vi "Main.vi"() -> ()   [LabVIEW 2017]
doc: "This sample project is built upon the standard state machine template and shows how you could create an application that acquires, analyzes, and presents data. It includes functionality for presenting configuration dialogs, preserving settings between executions, loading and saving data, as well as exporting graph images and text files.\n\nIt is most appropriate for data that is acquired instantly as it does not allow for screen updates mid acquisition nor does it allow for continuous streaming to disk."
uses:
  controls/State.ctl
  controls/UI References.ctl
  controls/Graph Data.ctl
  <vilib>/Utility/miscctls.llb/LVAnnotationListTypeDef.ctl
  <vilib>/Utility/miscctls.llb/LVCursorListTypeDef.ctl
  controls/User Specified Data.ctl
  controls/HW Configuration.ctl
  controls/Analysis Configuration.ctl
  controls/New Data Behavior.ctl
  controls/Signal Configuration.ctl
panel:
  in  "Settings":bool
  in  "Snapshot":bool
  in  "Analyze":bool
  in  "Clear":bool
  in  "Exit":bool
  in  "Acquire":bool
  in  "Export":bool
  in  "Save Data":bool
  in  "Load Data":bool
  in  "Tab Control":enum32{"Data", "FFT Magnitude", "FFT Phase"}(tab)
  out "Data Graph":waveform(dbl)[](graph)
  out "FFT Magnitude":cluster{"f0":dbl, "df":dbl, "magnitude":dbl[]}[](graph)
  out "FFT Phase":cluster{"f0":dbl, "df":dbl, "magnitude":dbl[]}[](graph)
  out "Status Bar":string
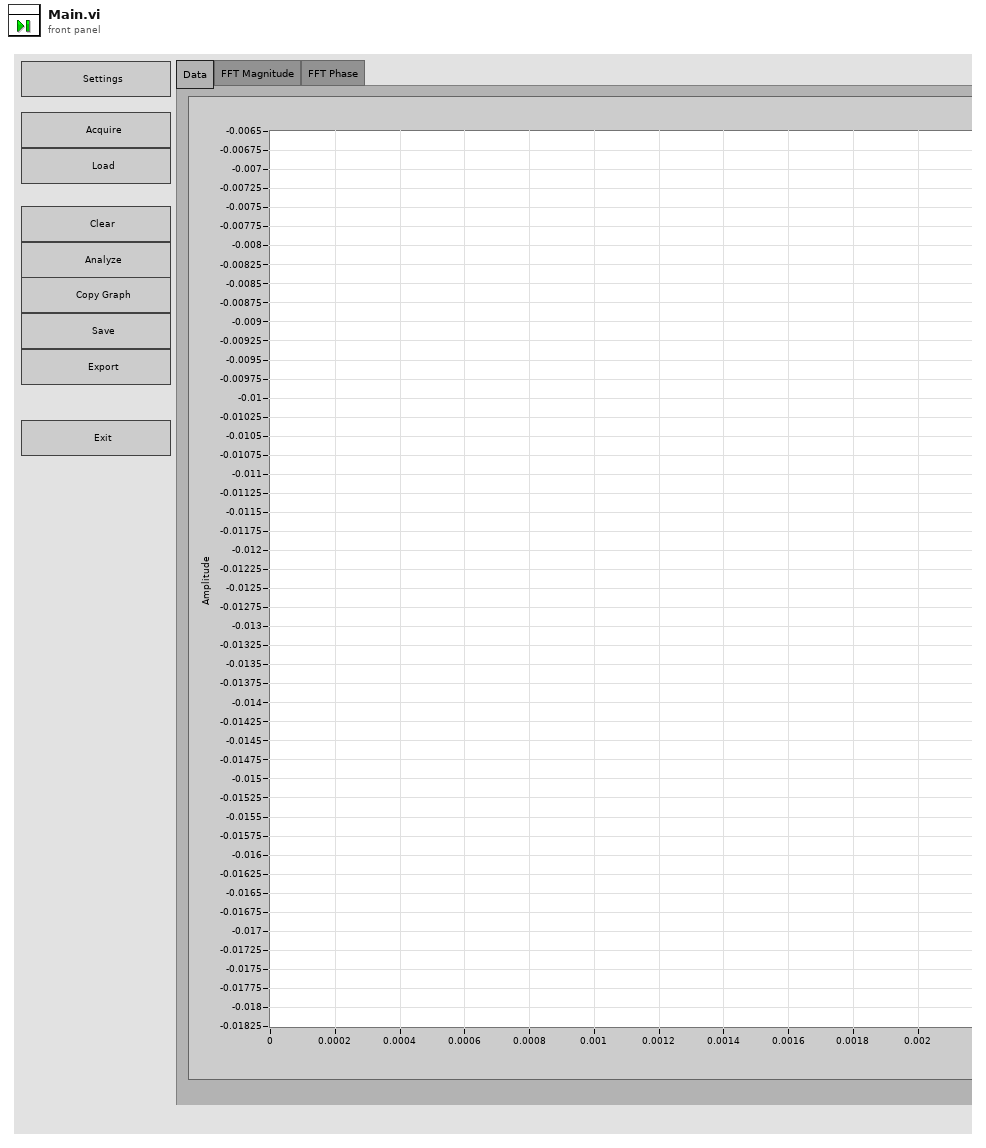
[diagram p1: front panel]
types:
  T1 = typedef "UI References.ctl" = cluster{"Stop Ref":refnum<vi>, "Save Ref":refnum<vi>, "Open Ref":refnum<vi>, "Export Ref":refnum<vi>, "Acquire Ref":refnum<vi>, "Configure Ref":refnum<vi>, "Graph Ref":refnum<vi>, "Clear Ref":refnum<vi>, "Analyze Ref":refnum<vi>, "Status Ref":refnum<vi>, "Snapshot Ref":refnum<vi>}
  T2 = typedef "Graph Data.ctl" = cluster{"Data":waveform(dbl)[], "Annotation List":T3, "Cursor List":T4, "Analysis Data":waveform(dbl)[]}
  T3 = typedef "LVAnnotationListTypeDef.ctl" = cluster{"Name":string, "Color":u32, "Style":u8, "Point Style":u8, "Name Visible":bool, "Allow Drag":bool, "Annotation Mode":u32, "Plot":i32, "Index":i32, "Position":cluster{"X":dbl, "Y":dbl}, "X Scale":u32, "Y Scale":u32, "Show Arrow":bool, "Lock Name":bool, "Plot Area":i32, "Label Offset":cluster{"X":dbl, "Y":dbl}}[]
  T4 = typedef "LVCursorListTypeDef.ctl" = cluster{"Name":string, "Color":u32, "Style":u8, "Point Style":u8, "Name Visible":bool, "Allow Drag":bool, "Cursor Mode":u32, "Plot":i32, "Index":i32, "Position":cluster{"X":dbl, "Y":dbl}, "X Scale":u32, "Y Scale":u32, "Watch Plots":i32[], "Watch All Plots":bool, "Plot Area":i32, "Label Offset":cluster{"X":dbl, "Y":dbl}}[]
  T5 = typedef "User Specified Data.ctl" = cluster{"Hardware Configuration":T6, "Analysis Configuration":T7, "Signal Type":enum16{"Single Chirp", "From Excel"}, "New Data Behavior":T8, "Signal Configuration":T9}
  T6 = typedef "HW Configuration.ctl" = cluster{"Signal Channel":tag, "Response Channel":tag, "Trigger Channel":tag, "Number of acquisitions":dbl}
  T7 = typedef "Analysis Configuration.ctl" = cluster{"Statistics":bool}
  T8 = typedef "New Data Behavior.ctl" = enum16{"Replace", "Overlay", "Append"}
  T9 = typedef "Signal Configuration.ctl" = cluster{"Chirp Amplitude":dbl, "I/O Limit":dbl, "Sample Rate":dbl, "Chirp Duration (s)":dbl, "Upper Frequency":dbl, "Lower Frequency":dbl, "Windowing":enum16{"None", "Exponential", "Flat top", "Hamming", "Hanning", "Kaiser-Bessel", "Rectangular"}}
  T10 = cluster{"UI References":T1, "Graph Data":T2, "User Specified":T5}
  T11 = typedef "State.ctl" = enum16{"Initialize", "Wait for Event", "Update UI", "Configure", "Acquire", "Load Data", "Save Data", "Clear Data", "Export Data", "Analyze", "Copy Graph", "Exit"}
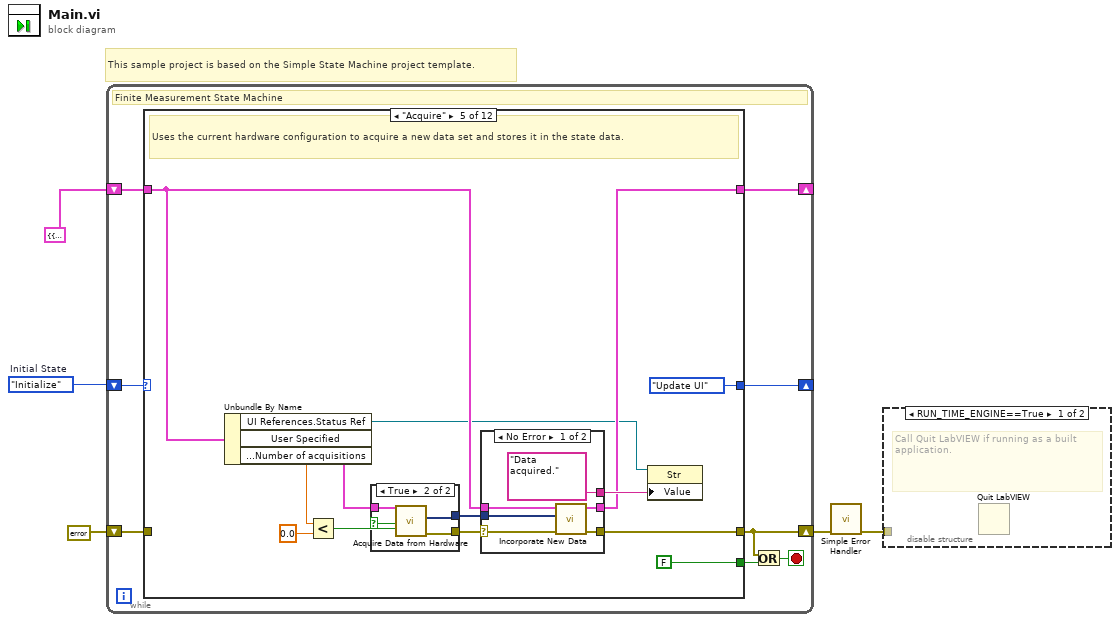
[diagram p0: block diagram]
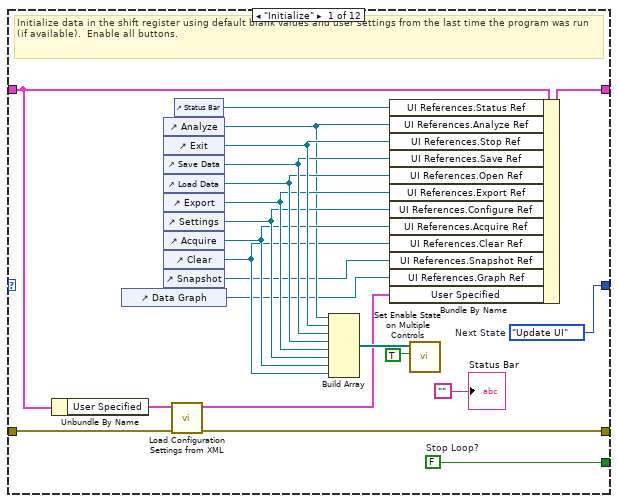
[diagram p3: hidden frame]
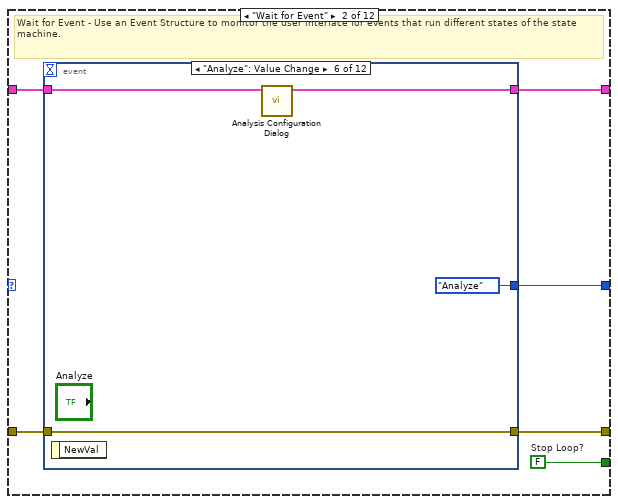
[diagram p4: hidden frame]
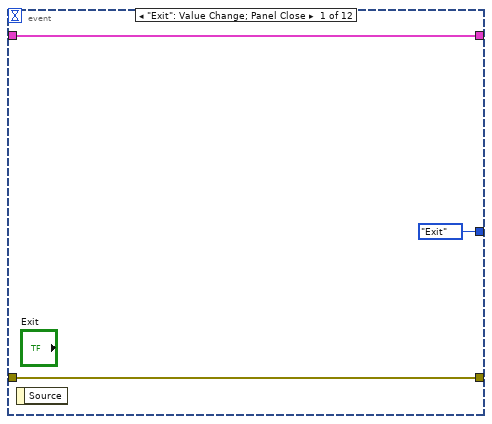
[diagram p5: hidden frame]
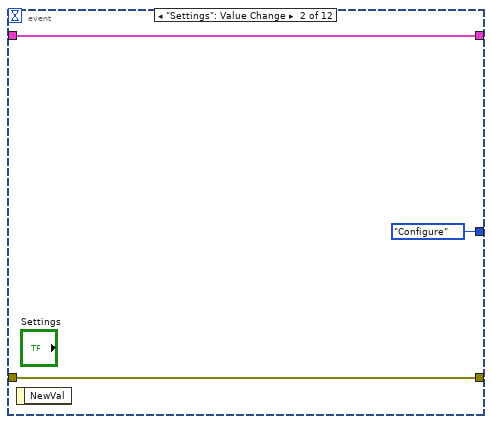
[diagram p6: hidden frame]
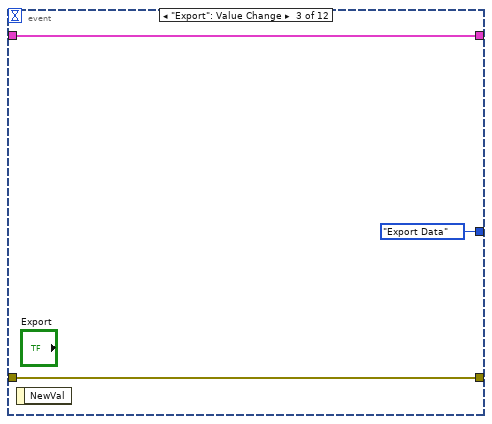
[diagram p7: hidden frame]
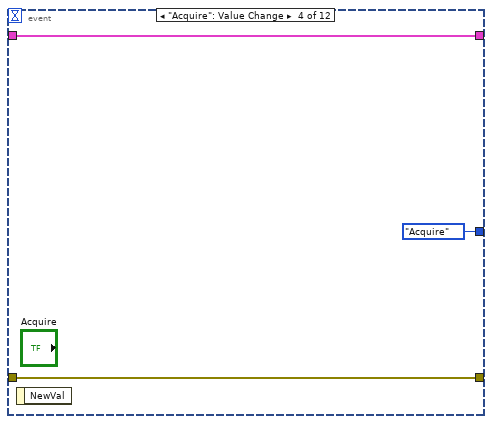
[diagram p8: hidden frame]
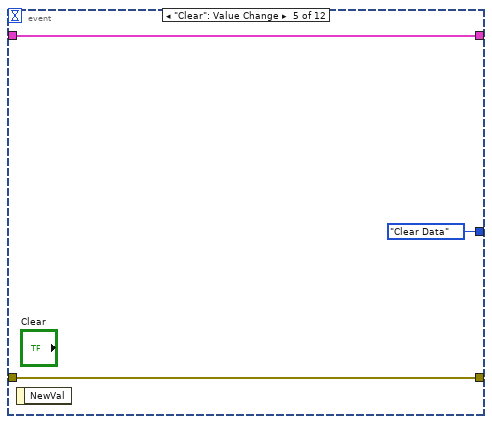
[diagram p9: hidden frame]
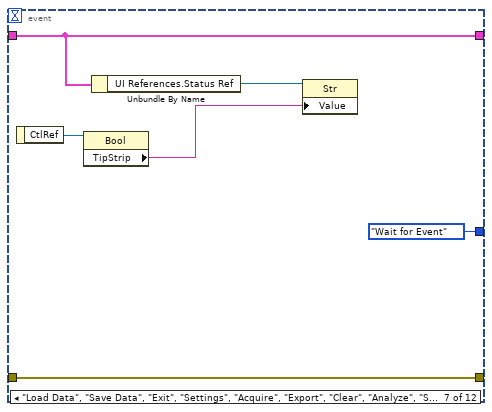
[diagram p10: hidden frame]
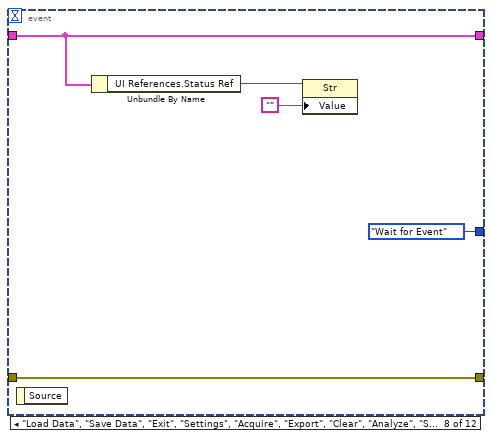
[diagram p11: hidden frame]
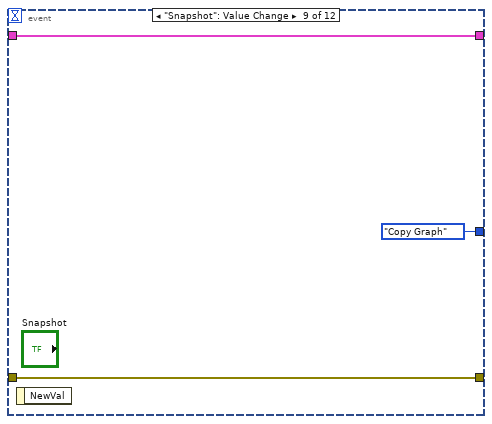
[diagram p12: hidden frame]
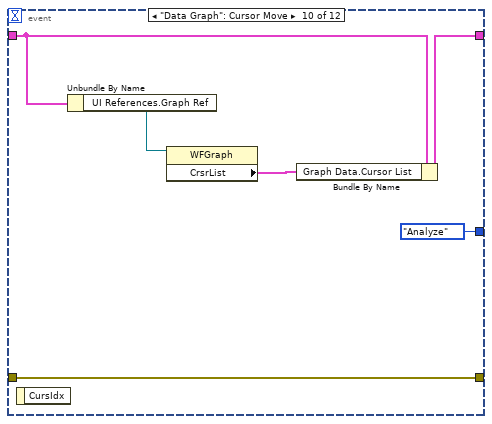
[diagram p13: hidden frame]
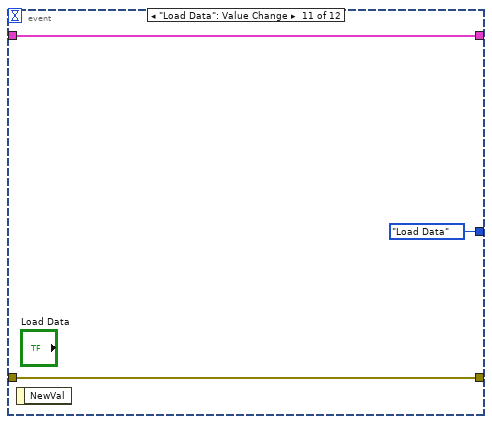
[diagram p14: hidden frame]
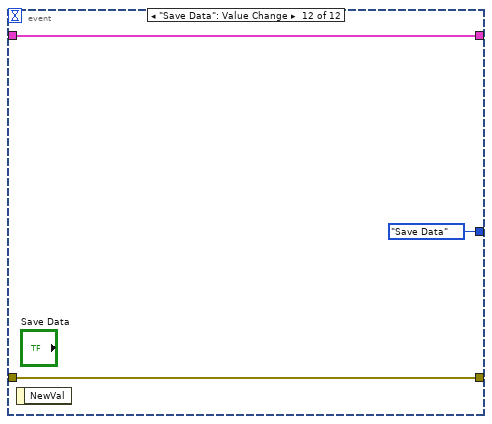
[diagram p15: hidden frame]
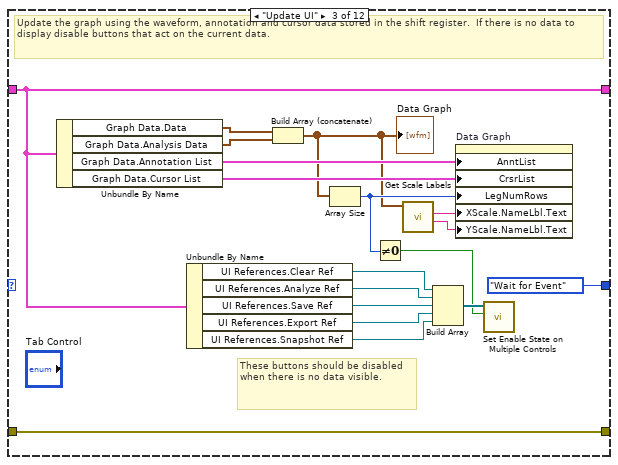
[diagram p16: hidden frame]
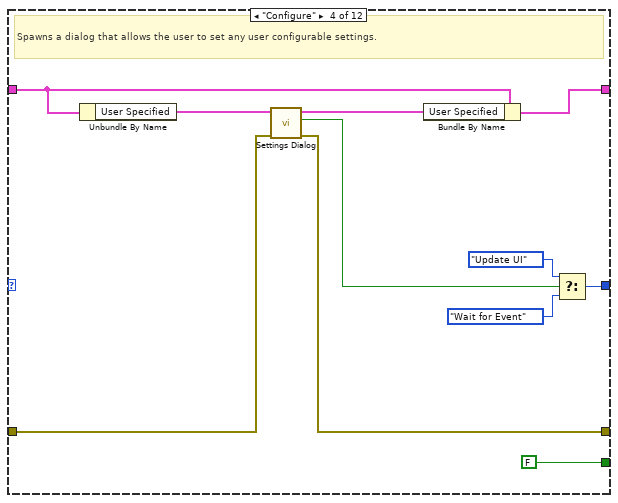
[diagram p17: hidden frame]
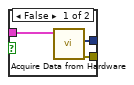
[diagram p18: hidden frame]
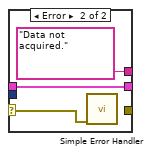
[diagram p19: hidden frame]
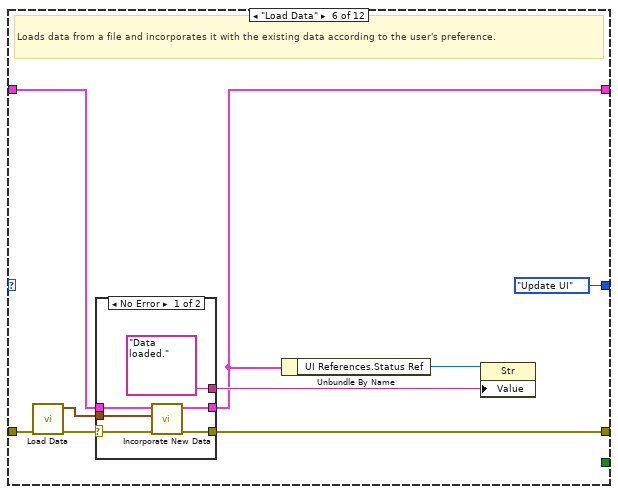
[diagram p20: hidden frame]
diagram:
  w5 = State."Initialize"  # Initial State
  # "This sample project is based on the Simple State Machine project template."
  n1 = while {
    shift-right: [w12] -> _
    shift-left: w5 -> [w13]
    shift-right: [w10] -> _
    shift-left: T10 {"UI References"={"Stop Ref"=refnum, "Save Ref"=refnum, "Open Ref"=refnum, "Export Ref"=refnum, "Acquire Ref"=refnum, "Configure Ref"=refnum, "Graph Ref"=refnum, "Clear Ref"=refnum, "Analyze Ref"=refnum, "Status Ref"=refnum, "Snapshot Ref"=refnum}, "Graph Data"={"Data"=[], "Annotation List"=[], "Cursor List"=[], "Analysis Data"=[]}, "User Specified"={"Hardware Configuration"={"Signal Channel"="", "Response Channel"="", "Trigger Channel"="", "Number of acquisitions"=0.0}, "Analysis Configuration"={"Statistics"=FALSE}, "Signal Type"=enum."Single Chirp", "New Data Behavior"=enum."Replace", "Signal Configuration"={"Chirp Amplitude"=0.1, "I/O Limit"=10.0, "Sample Rate"=1000000.0, "Chirp Duration (s)"=10000000.0, "Upper Frequency"=0.0, "Lower Frequency"=0.0, "Windowing"=enum."None"}}} ("Data") -> [w11]
    shift-right: [w6] -> w2
    shift-left: errorcluster {"status"=FALSE, "code"=0, "source"=""} ("error constant") -> [w9]
    stop <- w7 stop-if-true
    # "Finite Measurement State Machine"
    n2 = case shown="\"Acquire\"" w13 {
      tunnel: [w35 w41 State."Wait for Event" ("(Value Not Used)") w108 State."Update UI" ("Next State") State."Update UI" ("(Value Not Used)") State."Wait for Event" ("(Value Not Used)") State."Wait for Event" ("(Value Not Used)") State."Update UI" ("(Value Not Used)") State."Update UI" ("(Value Not Used)") State."Wait for Event" ("(Value Not Used)") w208] -> w12
      tunnel: [w34 w40 _ FALSE ("Stop Loop?") FALSE ("Stop Loop?") _ _ _ _ _ _ w207] -> w8
      tunnel: w11 -> [w25 w39 w101 w114 w124 w152 w165 w174 w187 w193 w197 w205]
      tunnel: [w33 w38 w101 w113 w123 w146 w165 w174 w186 w193 w197 w205] -> w10
      tunnel: w9 -> [w23 w37 w104 w112 _ w151 w167 w179 w189 w195 w199 w202]
      tunnel: [w22 w36 w104 w111 w119 w150 w163 w175 w189 w195 w198 w201] -> w6
      frame "Initialize" {
        w34 = FALSE  # Stop Loop?
        w35 = State."Update UI"  # Next State
        # "Initialize data in the shift register using default blank values and user settings from the last time the program was run (if available).  Enable all buttons."
        n3 = Unbundle By Name(w25) -> ("User Specified"=w24:T5)
        n4 = control-ref of="Data Graph"() -> (w14:refnum<vi>)
        n5 = control-ref of="Analyze"() -> (w21:refnum<vi>)
        n6 = control-ref of="Exit"() -> (w32:refnum<vi>)
        n7 = control-ref of="Save Data"() -> (w31:refnum<vi>)
        n8 = control-ref of="Load Data"() -> (w30:refnum<vi>)
        n9 = control-ref of="Export"() -> (w29:refnum<vi>)
        n10 = control-ref of="Settings"() -> (w28:refnum<vi>)
        n11 = control-ref of="Acquire"() -> (w27:refnum<vi>)
        n12 = control-ref of="Clear"() -> (w19:refnum<vi>)
        n13 = control-ref of="Snapshot"() -> (w15:refnum<vi>)
        n14 = call "Load Configuration Settings from XML.vi"("error in (no error)"=w23, "User Configuration in"=w24) -> ("error out"=w22:errorcluster, "User Configuration out"=w17:T5)  [unwired: 8 in]
        n15 = control-ref of="Status Bar"() -> (w20:refnum<vi>)
        n16 = Build Array(w21, w32, w31, w30, w29, w28, w27, w19) -> (w26:refnum<vi>[])
        n17 = Bundle By Name(cluster=w25, "UI References.Status Ref"=w20, "UI References.Analyze Ref"=w21, "UI References.Stop Ref"=w32, "UI References.Save Ref"=w31, "UI References.Open Ref"=w30, "UI References.Export Ref"=w29, "UI References.Configure Ref"=w28, "UI References.Acquire Ref"=w27, "UI References.Clear Ref"=w19, "UI References.Snapshot Ref"=w15, "UI References.Graph Ref"=w14, "User Specified"=w17) -> (w33:T10)
        n18 = call "Set Enable State on Multiple Controls.vi"("Enable?"=TRUE, "Controls"=w26) -> ()  [unwired: 10 in]
        "Status Bar" <- "" ("Status Bar")
      }
      frame "Wait for Event" {
        w40 = FALSE  # Stop Loop?
        # "Wait for Event - Use an Event Structure to monitor the user interface for events that run different states of the state machine."
        n19 = event shown="[5] \"Analyze\": Value Change" {
          selector: _ -> [_ _ _ _ _ _ _ _ _ _ _ _]
          dyn-events: _ -> [_ _ _ _ _ _ _ _ _ _ _ _]
          timeout: _ -> [_ _ _ _ _ _ _ _ _ _ _ _]
          tunnel: [State."Exit" ("Next State") State."Configure" ("Next State") State."Export Data" ("Next State") State."Acquire" ("Next State") State."Clear Data" ("Next State") State."Analyze" ("Next State") State."Wait for Event" ("Next State") State."Wait for Event" ("Next State") State."Copy Graph" ("Next State") State."Analyze" ("Next State") State."Load Data" ("Next State") State."Save Data" ("Next State")] -> w41
          tunnel: w39 -> [w43 w47 w50 w53 w56 w58 w64 w70 w74 w75 w82 w85]
          tunnel: [w43 w47 w50 w53 w56 w57 w64 w70 w74 w78 w82 w85] -> w38
          tunnel: w37 -> [w42 w46 w49 w52 w55 w60 w66 w71 w73 w80 w81 w84]
          tunnel: [w42 w46 w49 w52 w55 w60 w66 w71 w73 w80 w81 w84] -> w36
          event "Exit": Value Change; Panel Close {
            n20 = event-data() -> ()  [unwired: 1 in, 1 out]
          }
          event "Settings": Value Change {
            n21 = event-data() -> ()  [unwired: 1 in, 1 out]
          }
          event "Export": Value Change {
            n22 = event-data() -> ()  [unwired: 1 in, 1 out]
          }
          event "Acquire": Value Change {
            n23 = event-data() -> ()  [unwired: 1 in, 1 out]
          }
          event "Clear": Value Change {
            n24 = event-data() -> ()  [unwired: 1 in, 1 out]
          }
          event "Analyze": Value Change {
            n25 = event-data() -> ()  [unwired: 1 in, 1 out]
            n26 = call "Analysis Configuration Dialog.vi"("Data in"=w58) -> ("Data out"=w57:T10)  [unwired: 10 in]
          }
          event "Load Data", "Save Data", "Exit", "Settings", "Acquire", "Export", "Clear", "Analyze", "Snapshot": Mouse Enter {
            n27 = event-data() -> ("CtlRef"=w65:refnum<vi>)  [unwired: 1 in]
            n28 = property class="Bool"(reference=w65) -> ("TipStrip"=w62:string)  [unwired: 1 in, 2 out]
            n29 = Unbundle By Name(w64) -> ("UI References.Status Ref"=w63:refnum<vi>)
            n30 = property class="Str"(reference=w63, "Value"=w62) -> ()  [unwired: 1 in, 2 out]
          }
          event "Load Data", "Save Data", "Exit", "Settings", "Acquire", "Export", "Clear", "Analyze", "Snapshot": Mouse Leave {
            n31 = event-data() -> ()  [unwired: 1 in, 1 out]
            n32 = Unbundle By Name(w70) -> ("UI References.Status Ref"=w69:refnum<vi>)
            n33 = property class="Str"(reference=w69, "Value"="") -> ()  [unwired: 1 in, 2 out]
          }
          event "Snapshot": Value Change {
            n34 = event-data() -> ()  [unwired: 1 in, 1 out]
          }
          event "Data Graph": Cursor Move {
            n35 = event-data() -> ()  [unwired: 1 in, 1 out]
            n36 = Unbundle By Name(w75) -> ("UI References.Graph Ref"=w77:refnum<vi>)
            n37 = property class="WFGraph"(reference=w77) -> ("CrsrList"=w76:T4)  [unwired: 1 in, 2 out]
            n38 = Bundle By Name(cluster=w75, "Graph Data.Cursor List"=w76) -> (w78:T10)
          }
          event "Load Data": Value Change {
            n39 = event-data() -> ()  [unwired: 1 in, 1 out]
          }
          event "Save Data": Value Change {
            n40 = event-data() -> ()  [unwired: 1 in, 1 out]
          }
        }
      }
      frame "Update UI" {
        # "These buttons should be disabled when there is no data visible."
        # "Update the graph using the waveform, annotation and cursor data stored in the shift register.  If there is no data to display disable buttons that act on the current data."
        n41 = Unbundle By Name(w101) -> ("Graph Data.Data"=w97:waveform(dbl)[], "Graph Data.Analysis Data"=w87:waveform(dbl)[], "Graph Data.Annotation List"=w102:T3, "Graph Data.Cursor List"=w98:T4)
        n42 = Unbundle By Name(w101) -> ("UI References.Clear Ref"=w93:refnum<vi>, "UI References.Analyze Ref"=w92:refnum<vi>, "UI References.Save Ref"=w100:refnum<vi>, "UI References.Export Ref"=w90:refnum<vi>, "UI References.Snapshot Ref"=w91:refnum<vi>)
        n43 = Build Array (concatenate)(w97, w87) -> (w95:waveform(dbl)[])
        "Data Graph" <- w95
        n44 = Array Size(array=w95) -> (size(s)=w96:i32)
        n45 = Not Equal To 0?(x=w96) -> (x != 0?=w94:bool)
        n46 = call "Get Scale Labels.vi"("Array of Waveforms"=w95) -> ("Y Scale Label Text"=w88:string, "X Scale Label Text"=w89:string)  [unwired: 9 in]
        n47 = Build Array(w93, w92, w100, w90, w91) -> (w99:refnum<vi>[])
        n48 = property on="Data Graph" class="WFGraph (strict)"("AnntList"=w102, "CrsrList"=w98, "LegNumRows"=w96, "XScale.NameLbl.Text"=w89, "YScale.NameLbl.Text"=w88) -> ()  [unwired: 2 in, 2 out]
        n49 = call "Set Enable State on Multiple Controls.vi"("Enable?"=w94, "Controls"=w99) -> ()  [unwired: 10 in]
      }
      frame "Configure" {
        # "Spawns a dialog that allows the user to set any user configurable settings."
        n50 = Unbundle By Name(w114) -> ("User Specified"=w106:T5)
        n51 = call "Settings Dialog.vi"("error in (no error)"=w112, "User Specified Data in"=w106) -> ("error out"=w111:errorcluster, "UI Refresh Needed?"=w110:bool, "User specified data out"=w105:T5)  [unwired: 7 in]
        n52 = Bundle By Name(cluster=w114, "User Specified"=w105) -> (w113:T10)
        n53 = Select(t=State."Update UI" ("Next State if true"), s=w110, f=State."Wait for Event" ("Next State if false")) -> (s? t:f=w108:T11)
      }
      frame "Acquire" {
        # "Uses the current hardware configuration to acquire a new data set and stores it in the state data."
        n54 = Unbundle By Name(w124) -> ("UI References.Status Ref"=w120:refnum<vi>, "User Specified"=w126:T5, "User Specified.Hardware Configuration.Number of acquisitions"=w118:dbl)
        n55 = Less?(x=w118, y=0.0) -> (x < y?=w116:bool)
        n56 = case shown="True" w116 {
          tunnel: w126 -> [w131 w134]
          tunnel: [w130 w133] -> w122
          tunnel: [w129 w132] -> w121
          frame False {
            n57 = call "Acquire Data from Hardware.vi"("User Specified"=w131) -> ("error out"=w129:errorcluster, "Waveform Graph"=w130:dynamicdata)  [unwired: 8 in]
          }
          frame True {
            n58 = call "Acquire Data from Hardware.vi"("User Specified"=w134) -> ("error out"=w132:errorcluster, "Waveform Graph"=w133:dynamicdata)  [unwired: 8 in]
          }
        }
        n59 = case shown="No Error" w121 {
          selector: w121 -> [w137 w142]
          tunnel: w124 -> [w135 w143]
          tunnel: [w140 w143] -> w123
          tunnel: [w139 _] -> w119
          tunnel: w122 -> [w138 _]
          tunnel: ["Data acquired." ("Data acquired") "Data not acquired." ("Data not acquired")] -> w125
          frame No Error {
            n60 = call "Incorporate New Data.vi"("error in (no error)"=w137, "New Graph Data"=w138, "Data in"=w135) -> ("error out"=w139:errorcluster, "Data out"=w140:T10)  [unwired: 7 in]
          }
          frame Error {
            n61 = call <vilib>:"Simple Error Handler.vi"("error in (no error)"=w142) -> ()  [unwired: 4 in, 5 out]
          }
        }
        n62 = property class="Str"(reference=w120, "Value"=w125) -> ()  [unwired: 1 in, 2 out]
      }
      frame "Load Data" {
        # "Loads data from a file and incorporates it with the existing data according to the user's preference."
        n63 = call "Load Data.vi"("error in (no error)"=w151) -> ("error out"=w148:errorcluster, "New Graph Data"=w145:waveform(dbl)[])  [unwired: 9 in]
        n64 = case shown="No Error" w148 {
          selector: w148 -> [w155 w160]
          tunnel: w152 -> [w154 w161]
          tunnel: [w158 w161] -> w146
          tunnel: [w157 _] -> w150
          tunnel: w145 -> [w156 _]
          tunnel: ["Data loaded." ("Data loaded") "Data not loaded." ("Data not loaded")] -> w147
          frame No Error {
            n65 = call "Incorporate New Data.vi"("error in (no error)"=w155, "New Graph Data"=w156, "Data in"=w154) -> ("error out"=w157:errorcluster, "Data out"=w158:T10)  [unwired: 7 in]
          }
          frame Error {
            n66 = call <vilib>:"Simple Error Handler.vi"("error in (no error)"=w160) -> ()  [unwired: 4 in, 5 out]
          }
        }
        n67 = Unbundle By Name(w146) -> ("UI References.Status Ref"=w144:refnum<vi>)
        n68 = property class="Str"(reference=w144, "Value"=w147) -> ()  [unwired: 1 in, 2 out]
      }
      frame "Save Data" {
        # "Saves the existing measurement data to a file."
        n69 = Unbundle By Name(w165) -> ("UI References.Status Ref"=w164:refnum<vi>, "Graph Data.Data"=w168:waveform(dbl)[])
        n70 = call "Save Data.vi"("error in (no error)"=w167, "Data"=w168) -> ("error out"=w166:errorcluster)  [unwired: 9 in]
        n71 = case shown="No Error" w166 {
          selector: w166 -> [w170 w173]
          tunnel: ["Data saved." ("Data saved") "Data not saved." ("Data not saved")] -> w162
          tunnel: [w170 _] -> w163
          frame No Error {
          }
          frame Error {
            n72 = call <vilib>:"Simple Error Handler.vi"("error in (no error)"=w173) -> ()  [unwired: 4 in, 5 out]
          }
        }
        n73 = property class="Str"(reference=w164, "Value"=w162) -> ()  [unwired: 1 in, 2 out]
      }
      frame "Export Data" {
        # "Exports the currently loaded measurement and analysis data to a text file that can be imported into a spreadsheet or other application."
        n74 = Unbundle By Name(w174) -> ("UI References.Status Ref"=w176:refnum<vi>)
        n75 = call "Export Data.vi"("error in (no error)"=w179, "Data in"=w174) -> ("error out"=w177:errorcluster)  [unwired: 9 in]
        n76 = case shown="Error" w177 {
          selector: w177 -> [w181 w184]
          tunnel: ["Data exported." ("Data exported") "Data not exported." ("Data not exported")] -> w178
          tunnel: [w181 _] -> w175
          frame No Error {
          }
          frame Error {
            n77 = call <vilib>:"Simple Error Handler.vi"("error in (no error)"=w184) -> ()  [unwired: 4 in, 5 out]
          }
        }
        n78 = property class="Str"(reference=w176, "Value"=w178) -> ()  [unwired: 1 in, 2 out]
      }
      frame "Clear Data" {
        # "Clears the data currently in the graph."
        n79 = Bundle By Name(cluster=w187, "Graph Data"=T2 {"Data"=[], "Annotation List"=[], "Cursor List"=[], "Analysis Data"=[]} ("Graph")) -> (w186:T10)
      }
      frame "Analyze" {
        # "#CodeRecommended - add your own signal analysis here."
        # "Analyzes the measurement data using the user selected routines and adds annotations and calculated channels to the graph where appropriate."
        n80 = Unbundle By Name(w193) -> ("Graph Data"=w194:T2)
        n81 = call "Statistical Analysis.vi"("Graph Data In"=w194) -> ("FFT Phase"=→"FFT Phase":cluster{"f0":dbl, "df":dbl, "magnitude":dbl[]}[], "FFT Magnitude"=→"FFT Magnitude":cluster{"f0":dbl, "df":dbl, "magnitude":dbl[]}[])  [unwired: 6 in, 2 out]
        n82 = local write "Tab Control"(enum32{"Data", "FFT Magnitude", "FFT Phase"}."FFT Magnitude" ("Tab Control")) -> ()
      }
      frame "Copy Graph" {
        # "Places an image of the graph on the clipboard for pasting into reports or emails."
        n83 = call "Copy Graph to Clipboard.vi"("error in (no error)"=w199, "Graph Data"=w197) -> ("error out"=w198:errorcluster)  [unwired: 9 in]
      }
      frame "Exit" {
        w207 = TRUE  # Stop Loop?
        w208 = State."Exit"  # (Value Not Used)
        # "The state value is not used here since this is the last iteration of the state machine loop"
        # "Saves the user's settings to an XML file and stops execution."
        n84 = Unbundle By Name(w205) -> ("UI References.Status Ref"=w203:refnum<vi>, "User Specified"=w206:T5)
        n85 = call "Save Configuration Settings to XML.vi"("error in (no error)"=w202, "User Configuration"=w206) -> ("error out"=w201:errorcluster)  [unwired: 9 in]
        n86 = property class="Str"(reference=w203, "Value"="Stopped." ("Stopped")) -> ()  [unwired: 1 in, 2 out]
      }
    }
    n87 = Or(x=w6, y=w8) -> (x .or. y?=w7:bool)
  }
  n88 = call <vilib>:"Simple Error Handler.vi"("error in (no error)"=w2) -> ("error out"=w1:errorcluster)  [unwired: 4 in, 4 out]
  n89 = disable-structure shown="RUN_TIME_ENGINE==True" {
    disable-tunnel: w1 -> [_ _]
    frame condition #0 {
      # "Call Quit LabVIEW if running as a built application."
      n90 = Quit LabVIEW() -> ()  [unwired: 1 in]
    }
    frame condition #1 (active) {
    }
  }
